vi "Create Writer.vi"(8 "error in (no error)":errorcluster, 11 "Enclave in":refnum<class "Enclave.lvclass">) -> (0 "error out":errorcluster, 2 "Writer":refnum<class "Writer.lvclass">, 3 "Enclave out":refnum<class "Enclave.lvclass">)   [LabVIEW 2022 SP3, in "Enclave.lvlib" / "Enclave.lvclass"]
uses:
  Enclave.lvclass
  Writer/Writer.lvclass
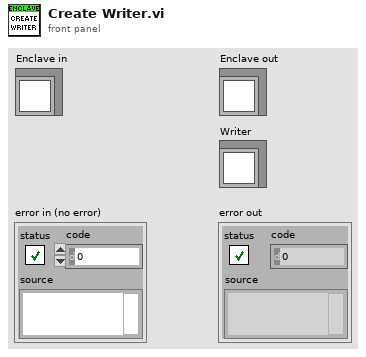
[diagram p1: front panel]
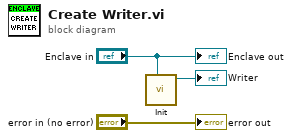
[diagram p0: block diagram]
diagram:
  n1 = call "Init.vi"("Enclave"="Enclave in") -> ("Writer out"=→"Writer":refnum<class "Writer.lvclass">)  [unwired: 9 in, 1 out]
  "error out" <- "error in (no error)"
  "Enclave out" <- "Enclave in"
